vi "Start Sync.vi"(8 "error in (no error)":errorcluster, 11 "gRPC Server in":refnum<class "GreeterService.lvclass">) -> (0 "error out":errorcluster, 3 "gRPC Server out":refnum<class "GreeterService.lvclass">)   [LabVIEW 2019, in "Generated_server.lvlib" / "GreeterService.lvclass"]
uses:
  GreeterService.lvclass
  GreeterService.lvclass/GreeterService.ctl
  RPC Messages/Greeter_res.ctl
  RPC Messages/Greeter_res_res_oneof/Greeter_res_res_oneof.lvclass
  RPC Messages/Greeter_req_req_oneof/Greeter_req_req_oneof.lvclass/Greeter_req_req_oneof.ctl
  RPC Messages/Greeter_MessageA.ctl
  RPC Messages/Greeter_MessageA_oneof_a/Greeter_MessageA_oneof_a.lvclass
  RPC Messages/Greeter_MessageA_oneof_a/Greeter_MessageA_oneof_a.lvclass/Greeter_MessageA_oneof_a.ctl
  RPC Messages/Greeter_res_res_oneof/Greeter_res_res_oneof.lvclass/Greeter_res_res_oneof.ctl
  Generated_server.lvlib
  RPC Messages/Greeter_req_req_oneof/Greeter_req_req_oneof.lvclass
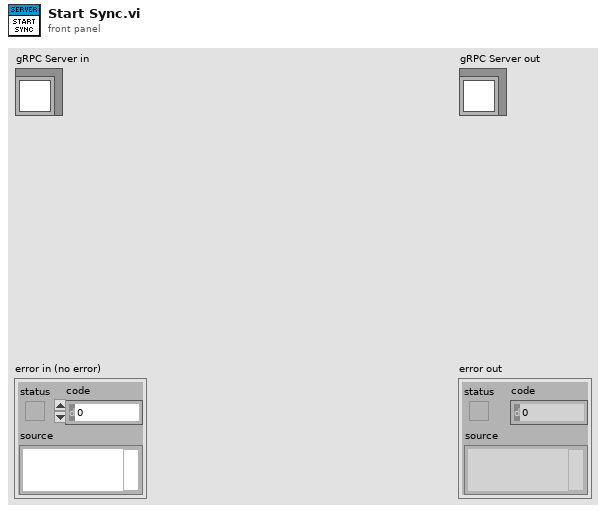
[diagram p1: front panel]
types:
  T1 = typedef "Generated_server.lvlib/Greeter_res.ctl" = cluster{"res_id":i32, "Greeter_res_res_oneof":refnum<class "Greeter_res_res_oneof.lvclass">}
  T2 = typedef "Generated_server.lvlib/Greeter_MessageA.ctl" = cluster{"Greeter_MessageA_oneof_a":refnum<class "Greeter_MessageA_oneof_a.lvclass">}
  T3 = typedef "Generated_server.lvlib/GreeterService.lvclass/Server Internal UEs.ctl" = cluster{"GreeterService GetFeature Internal UE":refnum<user-event>}
  T4 = typedef "Generated_server.lvlib/GreeterService.lvclass/Server gRPC UEs.ctl" = cluster{"GreeterService GetFeature gRPC UE":refnum<user-event>}
  T5 = typedef "grpc-lvsupport-release.lvlib/grpcId.ctl" = u64
  T6 = typedef "Generated_server.lvlib/Greeter_req.ctl" = cluster{"req_id":i32, "Greeter_req_req_oneof":refnum<class "Greeter_req_req_oneof.lvclass">}
  T7 = typedef "grpc-lvsupport.lvlib/grpcId.ctl" = u64
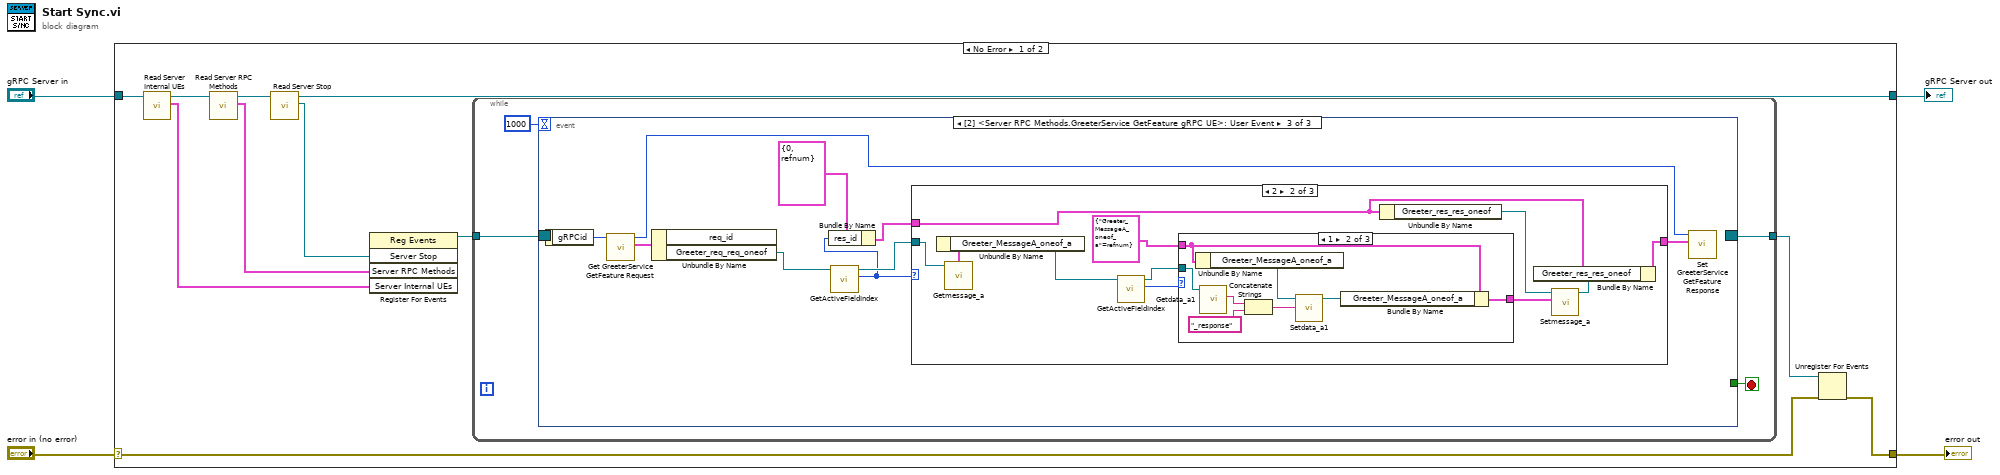
[diagram p0: block diagram]
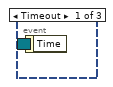
[diagram p2: hidden frame]
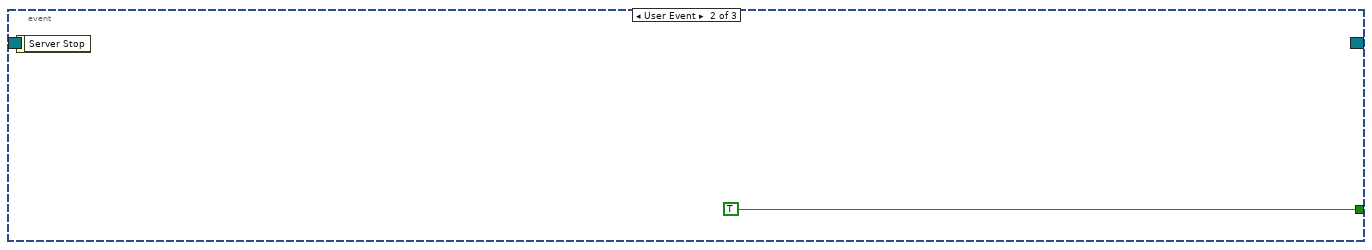
[diagram p3: hidden frame]
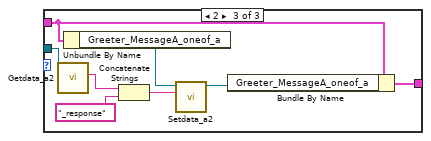
[diagram p6: hidden frame]
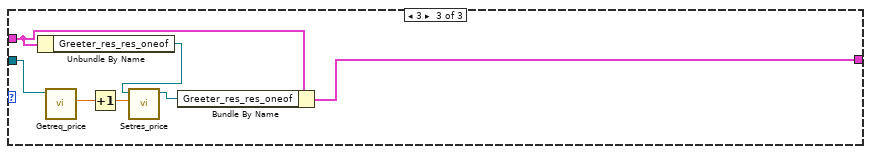
[diagram p7: hidden frame]
diagram:
  n1 = case shown="No Error" "error in (no error)" {
    selector: "error in (no error)" -> [w9 w67]
    tunnel: [w8 w67] -> w3
    tunnel: [w6 w66] -> w1
    tunnel: "gRPC Server in" -> [w15 w66]
    frame No Error {
      n2 = call "Read Server Internal UEs.vi"("SignalGeneratorService in"=w15) -> ("Server Internal UEs"=w13:T3, "SignalGeneratorService out"=w14:refnum<class "GreeterService.lvclass">)  [unwired: 8 in, 1 out]
      n3 = call "Read Server RPC Methods.vi"("SignalGeneratorService in"=w14) -> ("Server RPC Methods"=w7:T4, "SignalGeneratorService out"=w12:refnum<class "GreeterService.lvclass">)  [unwired: 8 in, 1 out]
      n4 = call-dynamic "Read Server Stop.vi"("iService in"=w12) -> ("Server Stop"=w5:refnum<user-event>, "iService out"=w6:refnum<class "GreeterService.lvclass">)  [unwired: 8 in, 1 out]
      n5 = register-events(w5, w7, w13) -> (reference out=w11:refnum<event-registration>)  [unwired: 2 in, 1 out]
      n6 = while {
        tunnel: w11 -> [w19]
        tunnel: [w17] -> w10
        stop <- w18 stop-if-true
        n7 = event "RPC Methods Event Structure" shown="[2] <Server RPC Methods.GreeterService GetFeature gRPC UE>: User Event" {
          selector: w19 -> [_ _ _]
          dyn-events: [_ _ _] -> w17
          timeout: 1000 -> [_ _ _]
          tunnel: [_ TRUE _] -> w18
          event Timeout {
            n8 = event-data() -> ()  [unwired: 1 in, 1 out]
          }
          event User Event {
            n9 = event-data() -> ()  [unwired: 1 in, 1 out]
          }
          event User Event {
            n10 = event-data() -> ("gRPCid"=w29:T5)  [unwired: 1 in]
            n11 = call "Get GreeterService GetFeature Request.vi"("gRPCid in"=w29) -> ("Message Data"=w28:T6, "gRPCid out"=w22:T7)  [unwired: 8 in, 1 out]
            n12 = Unbundle By Name(w28) -> ("Greeter_req_req_oneof"=w26:refnum<class "Greeter_req_req_oneof.lvclass">)  [unwired: 1 out]
            n13 = call "GetActiveFieldIndex.vi"("OneOfTemplate in"=w26) -> ("Active Field Index"=w21:i32, "OneOfTemplate out"=w25:refnum<class "Greeter_req_req_oneof.lvclass">)  [unwired: 8 in, 1 out]
            n14 = Bundle By Name(cluster=T1 {"res_id"=0, "Greeter_res_res_oneof"=refnum} ("Greeter_res"), "res_id"=w21) -> (w24:T1)
            n15 = case shown="2" w21 {
              tunnel: w25 -> [_ w36 w65]
              tunnel: w24 -> [w30 w33 w61]
              tunnel: [w30 w31 w59] -> w23
              frame 0, Default {
              }
              frame 2 {
                n16 = call "Getmessage_a.vi"("OneOfTemplate in"=w36) -> ("Get_Val"=w41:T2)  [unwired: 8 in, 2 out]
                n17 = Unbundle By Name(w41) -> ("Greeter_MessageA_oneof_a"=w40:refnum<class "Greeter_MessageA_oneof_a.lvclass">)
                n18 = call "GetActiveFieldIndex.vi"("OneOfTemplate in"=w40) -> ("Active Field Index"=w39:i32, "OneOfTemplate out"=w38:refnum<class "Greeter_MessageA_oneof_a.lvclass">)  [unwired: 8 in, 1 out]
                n19 = case shown="1" w39 {
                  tunnel: w38 -> [_ w50 w55]
                  tunnel: T2 {"Greeter_MessageA_oneof_a"=refnum} ("Greeter_MessageA") -> [w42 w45 w57]
                  tunnel: [w42 w43 w56] -> w35
                  frame 0, Default {
                  }
                  frame 1 {
                    n20 = Unbundle By Name(w45) -> ("Greeter_MessageA_oneof_a"=w46:refnum<class "Greeter_MessageA_oneof_a.lvclass">)
                    n21 = call "Getdata_a1.vi"("OneOfTemplate in"=w50) -> ("Get_Val"=w49:string)  [unwired: 8 in, 2 out]
                    n22 = Concatenate Strings(w49, "_response" ("string")) -> (w47:string)
                    n23 = call "Setdata_a1.vi"("Set_Val"=w47, "OneOfTemplate in"=w46) -> ("OneOfTemplate out"=w44:refnum<class "Greeter_MessageA_oneof_a.lvclass">)  [unwired: 8 in, 1 out]
                    n24 = Bundle By Name(cluster=w45, "Greeter_MessageA_oneof_a"=w44) -> (w43:T2)
                  }
                  frame 2 {
                    n25 = call "Getdata_a2.vi"("OneOfTemplate in"=w55) -> ("Get_Val"=w54:string)  [unwired: 8 in, 2 out]
                    n26 = Unbundle By Name(w57) -> ("Greeter_MessageA_oneof_a"=w51:refnum<class "Greeter_MessageA_oneof_a.lvclass">)
                    n27 = Concatenate Strings(w54, "_response" ("string")) -> (w52:string)
                    n28 = call "Setdata_a2.vi"("Set_Val"=w52, "OneOfTemplate in"=w51) -> ("OneOfTemplate out"=w53:refnum<class "Greeter_MessageA_oneof_a.lvclass">)  [unwired: 8 in, 1 out]
                    n29 = Bundle By Name(cluster=w57, "Greeter_MessageA_oneof_a"=w53) -> (w56:T2)
                  }
                }
                n30 = Unbundle By Name(w33) -> ("Greeter_res_res_oneof"=w34:refnum<class "Greeter_res_res_oneof.lvclass">)
                n31 = call "Setmessage_a.vi"("Set_Val"=w35, "OneOfTemplate in"=w34) -> ("OneOfTemplate out"=w32:refnum<class "Greeter_res_res_oneof.lvclass">)  [unwired: 8 in, 1 out]
                n32 = Bundle By Name(cluster=w33, "Greeter_res_res_oneof"=w32) -> (w31:T1)
              }
              frame 3 {
                n33 = Unbundle By Name(w61) -> ("Greeter_res_res_oneof"=w62:refnum<class "Greeter_res_res_oneof.lvclass">)
                n34 = call "Getreq_price.vi"("OneOfTemplate in"=w65) -> ("Get_Val"=w64:dbl)  [unwired: 8 in, 2 out]
                n35 = Increment(x=w64) -> (x+1=w63:dbl)
                n36 = call "Setres_price.vi"("Set_Val"=w63, "OneOfTemplate in"=w62) -> ("OneOfTemplate out"=w60:refnum<class "Greeter_res_res_oneof.lvclass">)  [unwired: 8 in, 1 out]
                n37 = Bundle By Name(cluster=w61, "Greeter_res_res_oneof"=w60) -> (w59:T1)
              }
            }
            n38 = call "Set GreeterService GetFeature Response.vi"("Message Data"=w23, "gRPCid in"=w22) -> ()  [unwired: 9 in, 1 out]
          }
        }
      }
      n39 = Unregister For Events(event registration refnum=w10, error in=w9) -> (error out=w8:errorcluster)
    }
    frame Error {
    }
  }
  "error out" <- w3
  "gRPC Server out" <- w1
